vi "Z900_navX_SERIAL_DecodePacket.vi"(8 "error (in)":errorcluster, 10 "Data (in)":u8[](array[numeric]), 11 "Packet (in)":string) -> (0 "error (out)":errorcluster, 1 "empty?":bool, 2 "Data":u8[](array[numeric]), 3 "Packet (out)":string)   [LabVIEW 2016]
uses:
  _TypeDefs/Z900_navX_DeviceRegisters.ctl
  _Util/Encode Protocol/Z900_navX_Util_EncodeProtocol_Int16.vi
  _Util/Z900_navX_Util_BigEndian_to_LittleEndian.vi
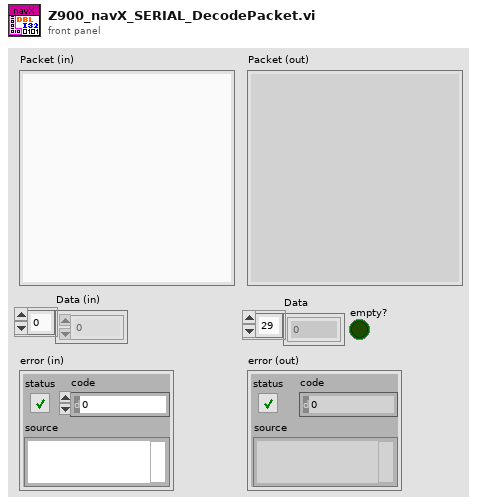
[diagram p1: front panel]
types:
  T1 = typedef "Z900_navX_DeviceRegisters.ctl" = u8
  T2 = cluster{"Device Register":T1, "index":i32, "length":i32}[]
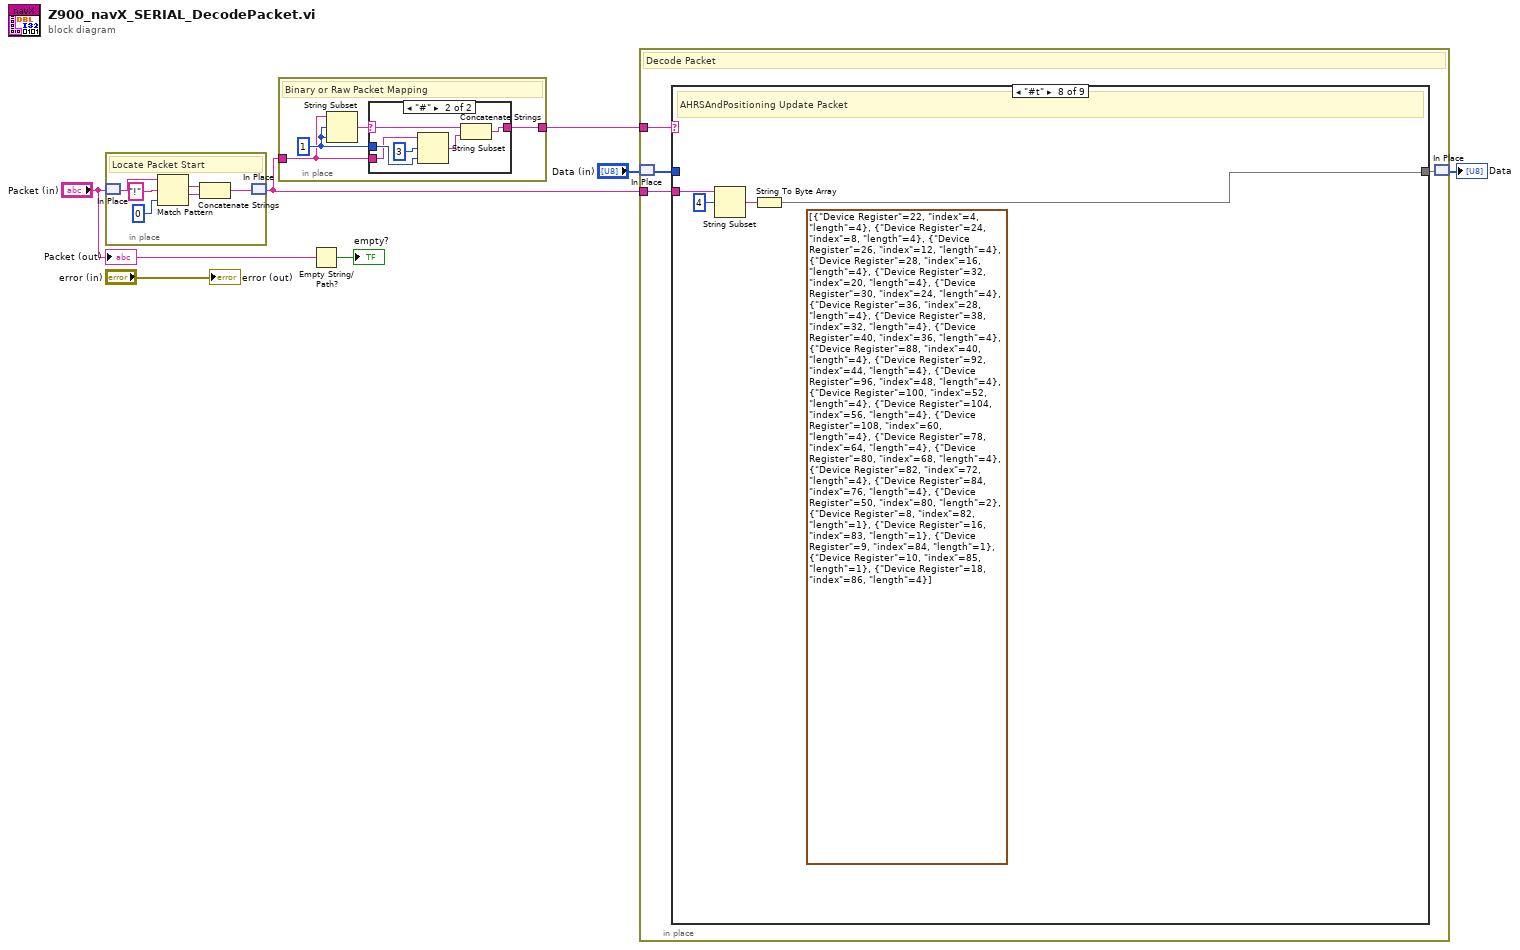
[diagram p0: block diagram]
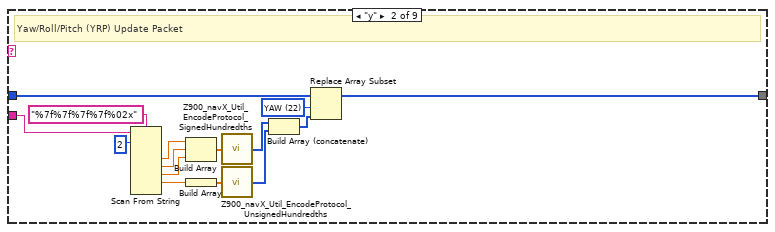
[diagram p3: hidden frame]
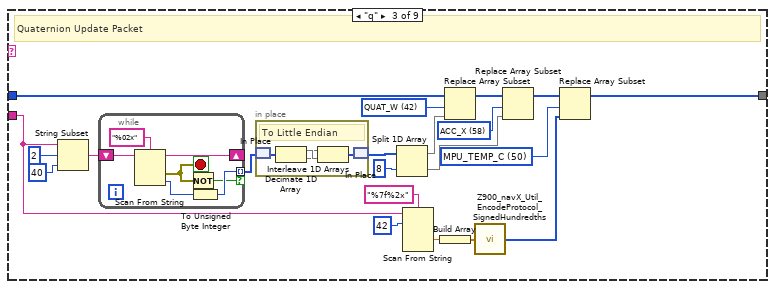
[diagram p4: hidden frame]
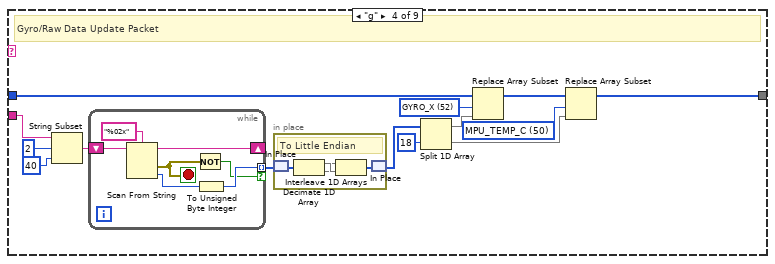
[diagram p5: hidden frame]
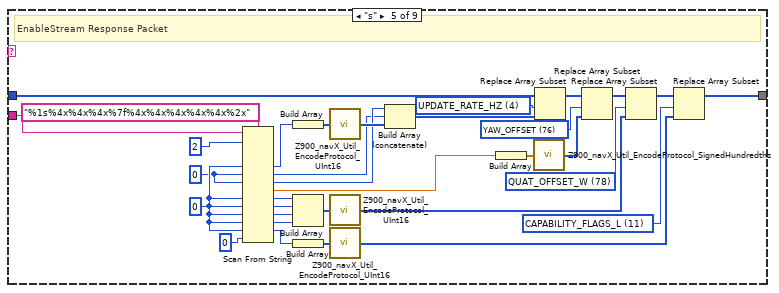
[diagram p6: hidden frame]
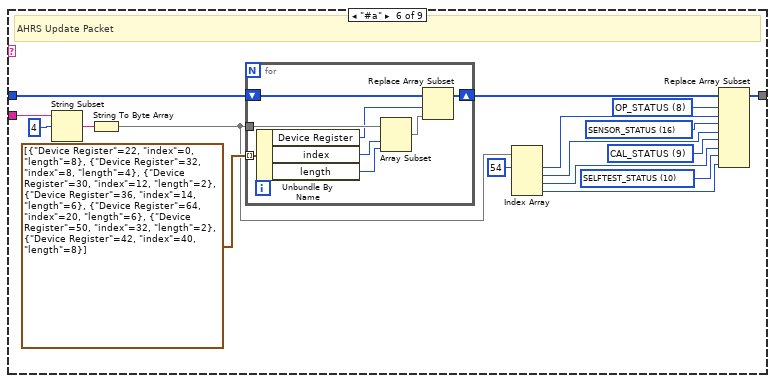
[diagram p7: hidden frame]
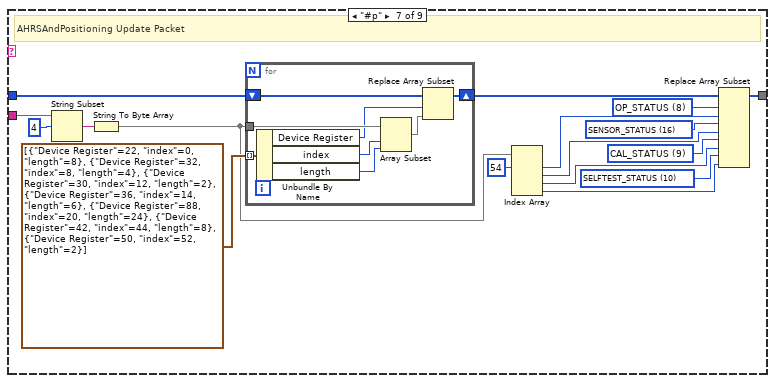
[diagram p8: hidden frame]
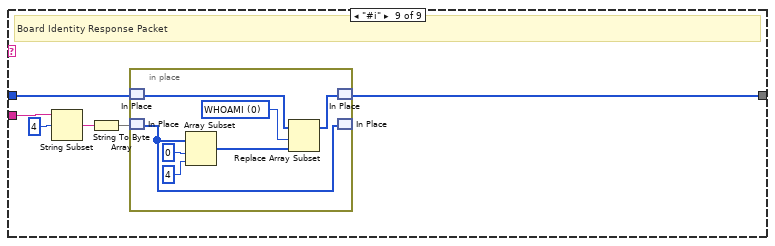
[diagram p9: hidden frame]
diagram:
  n1 = in-place {
    # "Locate Packet Start"
    n2 = in-place-match #1("Packet (in)") -> (w9:string)
    n3 = Match Pattern(string=w9, regular expression="!" ("Packet Start Char"), offset (0)=0 ("offset past match")) -> (match substring=w12:string, after substring=w11:string)  [unwired: 2 out]
    n4 = Concatenate Strings(w12, w11) -> (w8:string)
    n5 = in-place-match #1(w8) -> (w4:string)
  }
  n6 = in-place {
    in-place-border: w4 -> [w15]
    in-place-border: [w17] -> w5
    w16 = 1 ("length (rest)")
    # "Binary or Raw Packet Mapping"
    n7 = String Subset(string=w15, offset (0)=w16, length (rest)=w16) -> (substring=w14:string)
    n8 = case shown="\"#\"" w14 {
      selector: w14 -> [w18 w19]
      tunnel: [w18 w20] -> w17
      tunnel: w16 -> [_ w23]
      tunnel: w15 -> [_ w22]
      frame Default {
      }
      frame "#" {
        n9 = String Subset(string=w22, offset (0)=3, length (rest)=w23) -> (substring=w21:string)
        n10 = Concatenate Strings(w19, w21) -> (w20:string)
      }
    }
  }
  n11 = Empty String/Path?(string/path="Packet (in)") -> (empty?=→"empty?":bool)
  n12 = in-place {
    in-place-border: w5 -> [w28]
    in-place-border: w4 -> [w26]
    # "Decode Packet"
    n13 = in-place-match #2("Data (in)") -> (w27:u8[])
    n14 = case shown="\"#t\"" w28 {
      tunnel: w27 -> [w29 w35 w49 w86 w123 w137 w162 _ w190]
      tunnel: [w29 w30 w55 w79 w112 w135 w160 w185 w189] -> w25
      tunnel: w26 -> [_ w42 w60 w88 w129 w151 w161 w188 w192]
      frame Default {
        # "Unknown Packet"
      }
      frame "y" {
        w31 = T1 22 items=["WHOAMI"=0, "HW_REV"=1, "FW_VER_MAJOR"=2, "FW_VER_MINOR"=3, "UPDATE_RATE_HZ"=4, "ACCEL_FSR_G"=5, "GYRO_FSR_DPS"=6, "OP_STATUS"=8, "CAL_STATUS"=9, "SELFTEST_STATUS"=10, "CAPABILITY_FLAGS_L"=11, "CAPABILITY_FLAGS_H"=12, "SENSOR_STATUS"=16, "TIMESTAMP"=18, "YAW"=22, "ROLL"=24, "PITCH"=26, "HEADING"=28, "FUSED_HEADING"=30, "ALTITUDE_I"=32, "ALTITUDE_D"=34, "LINERA_ACC_X"=36, "LINERA_ACC_Y"=38, "LINERA_ACC_Z"=40, "QUAT_W"=42, "QUAT_X"=44, "QUAT_Y"=46, "QUAT_Z"=48, "MPU_TEMP_C"=50, "GYRO_X"=52, "GYRO_Y"=54, "GYRO_Z"=56, "ACC_X"=58, "ACC_Y"=60, "ACC_Z"=62, "MAG_X"=64, "MAG_Y"=66, "MAG_Z"=68, "PRESSURE_I"=70, "PRESSURE_D"=72, "PRESSURE_TEMP"=74, "YAW_OFFSET"=76, "QUAT_OFFSET_W"=78, "QUAT_OFFSET_X"=80, "QUAT_OFFSET_Y"=82, "QUAT_OFFSET_Z"=84, "INTEGRATION_CONTROL"=86, "VELOCITY_X"=88, "VELOCITY_Y"=92, "VELOCITY_Z"=96, "DISPLACMENT_X"=100, "DISPLACMENT_Y"=104, "DISPLACEMENT_Z"=108] ("Device Register")
        # "Yaw/Roll/Pitch (YRP) Update Packet"
        n15 = Scan From String(format string="%7f%7f%7f%7f%02x", input string=w42, initial scan location=2 ("offset (0)")) -> (output 1=w41:dbl, output 2=w40:dbl, output 3=w39:dbl, output 4=w37:dbl)  [unwired: 7 in, 3 out]
        n16 = Build Array(w41, w40, w39) -> (w38:dbl[])
        n17 = Build Array(w37) -> (w36:dbl[])
        n18 = call "Z900_navX_Util_EncodeProtocol_SignedHundredths.vi"("Signed Hundredths (0.00)"=w38) -> ("Little Endian"=w34:u8[])
        n19 = call "Z900_navX_Util_EncodeProtocol_UnsignedHundredths.vi"("Unsigned Hundredths (0.00)"=w36) -> ("Little Endian"=w33:u8[])
        n20 = Build Array (concatenate)(w34, w33) -> (w32:u8[])
        n21 = Replace Array Subset(array=w35, new element=w32, index=w31) -> (w30:u8[])
      }
      frame "q" {
        w45 = T1 42 items=["WHOAMI"=0, "HW_REV"=1, "FW_VER_MAJOR"=2, "FW_VER_MINOR"=3, "UPDATE_RATE_HZ"=4, "ACCEL_FSR_G"=5, "GYRO_FSR_DPS"=6, "OP_STATUS"=8, "CAL_STATUS"=9, "SELFTEST_STATUS"=10, "CAPABILITY_FLAGS_L"=11, "CAPABILITY_FLAGS_H"=12, "SENSOR_STATUS"=16, "TIMESTAMP"=18, "YAW"=22, "ROLL"=24, "PITCH"=26, "HEADING"=28, "FUSED_HEADING"=30, "ALTITUDE_I"=32, "ALTITUDE_D"=34, "LINERA_ACC_X"=36, "LINERA_ACC_Y"=38, "LINERA_ACC_Z"=40, "QUAT_W"=42, "QUAT_X"=44, "QUAT_Y"=46, "QUAT_Z"=48, "MPU_TEMP_C"=50, "GYRO_X"=52, "GYRO_Y"=54, "GYRO_Z"=56, "ACC_X"=58, "ACC_Y"=60, "ACC_Z"=62, "MAG_X"=64, "MAG_Y"=66, "MAG_Z"=68, "PRESSURE_I"=70, "PRESSURE_D"=72, "PRESSURE_TEMP"=74, "YAW_OFFSET"=76, "QUAT_OFFSET_W"=78, "QUAT_OFFSET_X"=80, "QUAT_OFFSET_Y"=82, "QUAT_OFFSET_Z"=84, "INTEGRATION_CONTROL"=86, "VELOCITY_X"=88, "VELOCITY_Y"=92, "VELOCITY_Z"=96, "DISPLACMENT_X"=100, "DISPLACMENT_Y"=104, "DISPLACEMENT_Z"=108] ("Device Register")
        w52 = T1 58 items=["WHOAMI"=0, "HW_REV"=1, "FW_VER_MAJOR"=2, "FW_VER_MINOR"=3, "UPDATE_RATE_HZ"=4, "ACCEL_FSR_G"=5, "GYRO_FSR_DPS"=6, "OP_STATUS"=8, "CAL_STATUS"=9, "SELFTEST_STATUS"=10, "CAPABILITY_FLAGS_L"=11, "CAPABILITY_FLAGS_H"=12, "SENSOR_STATUS"=16, "TIMESTAMP"=18, "YAW"=22, "ROLL"=24, "PITCH"=26, "HEADING"=28, "FUSED_HEADING"=30, "ALTITUDE_I"=32, "ALTITUDE_D"=34, "LINERA_ACC_X"=36, "LINERA_ACC_Y"=38, "LINERA_ACC_Z"=40, "QUAT_W"=42, "QUAT_X"=44, "QUAT_Y"=46, "QUAT_Z"=48, "MPU_TEMP_C"=50, "GYRO_X"=52, "GYRO_Y"=54, "GYRO_Z"=56, "ACC_X"=58, "ACC_Y"=60, "ACC_Z"=62, "MAG_X"=64, "MAG_Y"=66, "MAG_Z"=68, "PRESSURE_I"=70, "PRESSURE_D"=72, "PRESSURE_TEMP"=74, "YAW_OFFSET"=76, "QUAT_OFFSET_W"=78, "QUAT_OFFSET_X"=80, "QUAT_OFFSET_Y"=82, "QUAT_OFFSET_Z"=84, "INTEGRATION_CONTROL"=86, "VELOCITY_X"=88, "VELOCITY_Y"=92, "VELOCITY_Z"=96, "DISPLACMENT_X"=100, "DISPLACMENT_Y"=104, "DISPLACEMENT_Z"=108] ("Device Register")
        w57 = T1 50 items=["WHOAMI"=0, "HW_REV"=1, "FW_VER_MAJOR"=2, "FW_VER_MINOR"=3, "UPDATE_RATE_HZ"=4, "ACCEL_FSR_G"=5, "GYRO_FSR_DPS"=6, "OP_STATUS"=8, "CAL_STATUS"=9, "SELFTEST_STATUS"=10, "CAPABILITY_FLAGS_L"=11, "CAPABILITY_FLAGS_H"=12, "SENSOR_STATUS"=16, "TIMESTAMP"=18, "YAW"=22, "ROLL"=24, "PITCH"=26, "HEADING"=28, "FUSED_HEADING"=30, "ALTITUDE_I"=32, "ALTITUDE_D"=34, "LINERA_ACC_X"=36, "LINERA_ACC_Y"=38, "LINERA_ACC_Z"=40, "QUAT_W"=42, "QUAT_X"=44, "QUAT_Y"=46, "QUAT_Z"=48, "MPU_TEMP_C"=50, "GYRO_X"=52, "GYRO_Y"=54, "GYRO_Z"=56, "ACC_X"=58, "ACC_Y"=60, "ACC_Z"=62, "MAG_X"=64, "MAG_Y"=66, "MAG_Z"=68, "PRESSURE_I"=70, "PRESSURE_D"=72, "PRESSURE_TEMP"=74, "YAW_OFFSET"=76, "QUAT_OFFSET_W"=78, "QUAT_OFFSET_X"=80, "QUAT_OFFSET_Y"=82, "QUAT_OFFSET_Z"=84, "INTEGRATION_CONTROL"=86, "VELOCITY_X"=88, "VELOCITY_Y"=92, "VELOCITY_Z"=96, "DISPLACMENT_X"=100, "DISPLACMENT_Y"=104, "DISPLACEMENT_Z"=108] ("Device Register")
        # "Quaternion Update Packet"
        n22 = String Subset(string=w60, offset (0)=2, length (rest)=40 ("length (rest)")) -> (substring=w62:string)
        n23 = while {
          shift-right: [w74] -> _
          shift-left: w62 -> [w75]
          tunnel: [w72] -> w51 mode=indexing if=w70
          stop <- w71 stop-if-true
          n24 = Scan From String(format string="%02x", input string=w75) -> (remaining string=w74:string, error out=w71:errorcluster, output 1=w73:u32)  [unwired: 3 in, 1 out]
          n25 = Not(x=w71) -> (.not. x?=w70:bool)
          n26 = To Unsigned Byte Integer(number=w73) -> (unsigned 8bit integer=w72:u8)
        }
        n27 = in-place {
          # "To Little Endian"
          n28 = in-place-match #3(w51) -> (w67:u8[])
          n29 = Decimate 1D Array(w67) -> (w69:u8[], w68:u8[])
          n30 = Interleave 1D Arrays(w68, w69) -> (w66:u8[])
          n31 = in-place-match #3(w66) -> (w50:u8[])
        }
        n32 = Split 1D Array(array=w50, index=8) -> (first subarray=w47:u8[], second subarray=w46:u8[])
        n33 = Scan From String(format string="%7f%2x", input string=w60, initial scan location=u32 42) -> (output 1=w58:dbl)  [unwired: 4 in, 3 out]
        n34 = Build Array(w58) -> (w59:dbl[])
        n35 = Replace Array Subset(array=w49, new element=w47, index=w45) -> (w48:u8[])
        n36 = call "Z900_navX_Util_EncodeProtocol_SignedHundredths.vi"("Signed Hundredths (0.00)"=w59) -> ("Little Endian"=w56:u8[])
        n37 = Replace Array Subset(array=w48, new element=w46, index=w52) -> (w53:u8[])
        n38 = Replace Array Subset(array=w53, new element=w56, index=w57) -> (w55:u8[])
      }
      frame "g" {
        w81 = T1 50 items=["WHOAMI"=0, "HW_REV"=1, "FW_VER_MAJOR"=2, "FW_VER_MINOR"=3, "UPDATE_RATE_HZ"=4, "ACCEL_FSR_G"=5, "GYRO_FSR_DPS"=6, "OP_STATUS"=8, "CAL_STATUS"=9, "SELFTEST_STATUS"=10, "CAPABILITY_FLAGS_L"=11, "CAPABILITY_FLAGS_H"=12, "SENSOR_STATUS"=16, "TIMESTAMP"=18, "YAW"=22, "ROLL"=24, "PITCH"=26, "HEADING"=28, "FUSED_HEADING"=30, "ALTITUDE_I"=32, "ALTITUDE_D"=34, "LINERA_ACC_X"=36, "LINERA_ACC_Y"=38, "LINERA_ACC_Z"=40, "QUAT_W"=42, "QUAT_X"=44, "QUAT_Y"=46, "QUAT_Z"=48, "MPU_TEMP_C"=50, "GYRO_X"=52, "GYRO_Y"=54, "GYRO_Z"=56, "ACC_X"=58, "ACC_Y"=60, "ACC_Z"=62, "MAG_X"=64, "MAG_Y"=66, "MAG_Z"=68, "PRESSURE_I"=70, "PRESSURE_D"=72, "PRESSURE_TEMP"=74, "YAW_OFFSET"=76, "QUAT_OFFSET_W"=78, "QUAT_OFFSET_X"=80, "QUAT_OFFSET_Y"=82, "QUAT_OFFSET_Z"=84, "INTEGRATION_CONTROL"=86, "VELOCITY_X"=88, "VELOCITY_Y"=92, "VELOCITY_Z"=96, "DISPLACMENT_X"=100, "DISPLACMENT_Y"=104, "DISPLACEMENT_Z"=108] ("Device Register")
        w85 = T1 52 items=["WHOAMI"=0, "HW_REV"=1, "FW_VER_MAJOR"=2, "FW_VER_MINOR"=3, "UPDATE_RATE_HZ"=4, "ACCEL_FSR_G"=5, "GYRO_FSR_DPS"=6, "OP_STATUS"=8, "CAL_STATUS"=9, "SELFTEST_STATUS"=10, "CAPABILITY_FLAGS_L"=11, "CAPABILITY_FLAGS_H"=12, "SENSOR_STATUS"=16, "TIMESTAMP"=18, "YAW"=22, "ROLL"=24, "PITCH"=26, "HEADING"=28, "FUSED_HEADING"=30, "ALTITUDE_I"=32, "ALTITUDE_D"=34, "LINERA_ACC_X"=36, "LINERA_ACC_Y"=38, "LINERA_ACC_Z"=40, "QUAT_W"=42, "QUAT_X"=44, "QUAT_Y"=46, "QUAT_Z"=48, "MPU_TEMP_C"=50, "GYRO_X"=52, "GYRO_Y"=54, "GYRO_Z"=56, "ACC_X"=58, "ACC_Y"=60, "ACC_Z"=62, "MAG_X"=64, "MAG_Y"=66, "MAG_Z"=68, "PRESSURE_I"=70, "PRESSURE_D"=72, "PRESSURE_TEMP"=74, "YAW_OFFSET"=76, "QUAT_OFFSET_W"=78, "QUAT_OFFSET_X"=80, "QUAT_OFFSET_Y"=82, "QUAT_OFFSET_Z"=84, "INTEGRATION_CONTROL"=86, "VELOCITY_X"=88, "VELOCITY_Y"=92, "VELOCITY_Z"=96, "DISPLACMENT_X"=100, "DISPLACMENT_Y"=104, "DISPLACEMENT_Z"=108] ("Device Register")
        # "Gyro/Raw Data Update Packet"
        n39 = String Subset(string=w88, offset (0)=2, length (rest)=40 ("length (rest)")) -> (substring=w87:string)
        n40 = while {
          shift-right: [w99] -> _
          shift-left: w87 -> [w100]
          tunnel: [w97] -> w78 mode=indexing if=w95
          stop <- w96 stop-if-true
          n41 = Scan From String(format string="%02x", input string=w100) -> (remaining string=w99:string, error out=w96:errorcluster, output 1=w98:u32)  [unwired: 3 in, 1 out]
          n42 = Not(x=w96) -> (.not. x?=w95:bool)
          n43 = To Unsigned Byte Integer(number=w98) -> (unsigned 8bit integer=w97:u8)
        }
        n44 = in-place {
          # "To Little Endian"
          n45 = in-place-match #4(w78) -> (w92:u8[])
          n46 = Decimate 1D Array(w92) -> (w94:u8[], w93:u8[])
          n47 = Interleave 1D Arrays(w93, w94) -> (w91:u8[])
          n48 = in-place-match #4(w91) -> (w77:u8[])
        }
        n49 = Split 1D Array(array=w77, index=18) -> (first subarray=w84:u8[], second subarray=w80:u8[])
        n50 = Replace Array Subset(array=w86, new element=w84, index=w85) -> (w82:u8[])
        n51 = Replace Array Subset(array=w82, new element=w80, index=w81) -> (w79:u8[])
      }
      frame "s" {
        w105 = u8 0 ("default value 2")
        w114 = T1 11 items=["WHOAMI"=0, "HW_REV"=1, "FW_VER_MAJOR"=2, "FW_VER_MINOR"=3, "UPDATE_RATE_HZ"=4, "ACCEL_FSR_G"=5, "GYRO_FSR_DPS"=6, "OP_STATUS"=8, "CAL_STATUS"=9, "SELFTEST_STATUS"=10, "CAPABILITY_FLAGS_L"=11, "CAPABILITY_FLAGS_H"=12, "SENSOR_STATUS"=16, "TIMESTAMP"=18, "YAW"=22, "ROLL"=24, "PITCH"=26, "HEADING"=28, "FUSED_HEADING"=30, "ALTITUDE_I"=32, "ALTITUDE_D"=34, "LINERA_ACC_X"=36, "LINERA_ACC_Y"=38, "LINERA_ACC_Z"=40, "QUAT_W"=42, "QUAT_X"=44, "QUAT_Y"=46, "QUAT_Z"=48, "MPU_TEMP_C"=50, "GYRO_X"=52, "GYRO_Y"=54, "GYRO_Z"=56, "ACC_X"=58, "ACC_Y"=60, "ACC_Z"=62, "MAG_X"=64, "MAG_Y"=66, "MAG_Z"=68, "PRESSURE_I"=70, "PRESSURE_D"=72, "PRESSURE_TEMP"=74, "YAW_OFFSET"=76, "QUAT_OFFSET_W"=78, "QUAT_OFFSET_X"=80, "QUAT_OFFSET_Y"=82, "QUAT_OFFSET_Z"=84, "INTEGRATION_CONTROL"=86, "VELOCITY_X"=88, "VELOCITY_Y"=92, "VELOCITY_Z"=96, "DISPLACMENT_X"=100, "DISPLACMENT_Y"=104, "DISPLACEMENT_Z"=108] ("Device Register")
        w117 = T1 78 items=["WHOAMI"=0, "HW_REV"=1, "FW_VER_MAJOR"=2, "FW_VER_MINOR"=3, "UPDATE_RATE_HZ"=4, "ACCEL_FSR_G"=5, "GYRO_FSR_DPS"=6, "OP_STATUS"=8, "CAL_STATUS"=9, "SELFTEST_STATUS"=10, "CAPABILITY_FLAGS_L"=11, "CAPABILITY_FLAGS_H"=12, "SENSOR_STATUS"=16, "TIMESTAMP"=18, "YAW"=22, "ROLL"=24, "PITCH"=26, "HEADING"=28, "FUSED_HEADING"=30, "ALTITUDE_I"=32, "ALTITUDE_D"=34, "LINERA_ACC_X"=36, "LINERA_ACC_Y"=38, "LINERA_ACC_Z"=40, "QUAT_W"=42, "QUAT_X"=44, "QUAT_Y"=46, "QUAT_Z"=48, "MPU_TEMP_C"=50, "GYRO_X"=52, "GYRO_Y"=54, "GYRO_Z"=56, "ACC_X"=58, "ACC_Y"=60, "ACC_Z"=62, "MAG_X"=64, "MAG_Y"=66, "MAG_Z"=68, "PRESSURE_I"=70, "PRESSURE_D"=72, "PRESSURE_TEMP"=74, "YAW_OFFSET"=76, "QUAT_OFFSET_W"=78, "QUAT_OFFSET_X"=80, "QUAT_OFFSET_Y"=82, "QUAT_OFFSET_Z"=84, "INTEGRATION_CONTROL"=86, "VELOCITY_X"=88, "VELOCITY_Y"=92, "VELOCITY_Z"=96, "DISPLACMENT_X"=100, "DISPLACMENT_Y"=104, "DISPLACEMENT_Z"=108] ("Device Register")
        w120 = T1 76 items=["WHOAMI"=0, "HW_REV"=1, "FW_VER_MAJOR"=2, "FW_VER_MINOR"=3, "UPDATE_RATE_HZ"=4, "ACCEL_FSR_G"=5, "GYRO_FSR_DPS"=6, "OP_STATUS"=8, "CAL_STATUS"=9, "SELFTEST_STATUS"=10, "CAPABILITY_FLAGS_L"=11, "CAPABILITY_FLAGS_H"=12, "SENSOR_STATUS"=16, "TIMESTAMP"=18, "YAW"=22, "ROLL"=24, "PITCH"=26, "HEADING"=28, "FUSED_HEADING"=30, "ALTITUDE_I"=32, "ALTITUDE_D"=34, "LINERA_ACC_X"=36, "LINERA_ACC_Y"=38, "LINERA_ACC_Z"=40, "QUAT_W"=42, "QUAT_X"=44, "QUAT_Y"=46, "QUAT_Z"=48, "MPU_TEMP_C"=50, "GYRO_X"=52, "GYRO_Y"=54, "GYRO_Z"=56, "ACC_X"=58, "ACC_Y"=60, "ACC_Z"=62, "MAG_X"=64, "MAG_Y"=66, "MAG_Z"=68, "PRESSURE_I"=70, "PRESSURE_D"=72, "PRESSURE_TEMP"=74, "YAW_OFFSET"=76, "QUAT_OFFSET_W"=78, "QUAT_OFFSET_X"=80, "QUAT_OFFSET_Y"=82, "QUAT_OFFSET_Z"=84, "INTEGRATION_CONTROL"=86, "VELOCITY_X"=88, "VELOCITY_Y"=92, "VELOCITY_Z"=96, "DISPLACMENT_X"=100, "DISPLACMENT_Y"=104, "DISPLACEMENT_Z"=108] ("Device Register")
        w122 = T1 4 items=["WHOAMI"=0, "HW_REV"=1, "FW_VER_MAJOR"=2, "FW_VER_MINOR"=3, "UPDATE_RATE_HZ"=4, "ACCEL_FSR_G"=5, "GYRO_FSR_DPS"=6, "OP_STATUS"=8, "CAL_STATUS"=9, "SELFTEST_STATUS"=10, "CAPABILITY_FLAGS_L"=11, "CAPABILITY_FLAGS_H"=12, "SENSOR_STATUS"=16, "TIMESTAMP"=18, "YAW"=22, "ROLL"=24, "PITCH"=26, "HEADING"=28, "FUSED_HEADING"=30, "ALTITUDE_I"=32, "ALTITUDE_D"=34, "LINERA_ACC_X"=36, "LINERA_ACC_Y"=38, "LINERA_ACC_Z"=40, "QUAT_W"=42, "QUAT_X"=44, "QUAT_Y"=46, "QUAT_Z"=48, "MPU_TEMP_C"=50, "GYRO_X"=52, "GYRO_Y"=54, "GYRO_Z"=56, "ACC_X"=58, "ACC_Y"=60, "ACC_Z"=62, "MAG_X"=64, "MAG_Y"=66, "MAG_Z"=68, "PRESSURE_I"=70, "PRESSURE_D"=72, "PRESSURE_TEMP"=74, "YAW_OFFSET"=76, "QUAT_OFFSET_W"=78, "QUAT_OFFSET_X"=80, "QUAT_OFFSET_Y"=82, "QUAT_OFFSET_Z"=84, "INTEGRATION_CONTROL"=86, "VELOCITY_X"=88, "VELOCITY_Y"=92, "VELOCITY_Z"=96, "DISPLACMENT_X"=100, "DISPLACMENT_Y"=104, "DISPLACEMENT_Z"=108] ("Device Register")
        w106 = u16 0
        # "EnableStream Response Packet"
        n52 = Scan From String(format string="%1s%4x%4x%4x%7f%4x%4x%4x%4x%4x%2x", input string=w129, initial scan location=u32 2, default 2=w106, default 3=w105, default 4=w105, default 6=w106, default 7=w106, default 8=w106, default 9=w106, default 10=w106, default 11=u8 0) -> (output 2=w107:u16, output 3=w102:u8, output 4=w103:u8, output 5=w131:dbl, output 6=w128:u16, output 7=w127:u16, output 8=w126:u16, output 9=w125:u16, output 10=w111:u16)  [unwired: 5 in, 3 out]
        n53 = Build Array(w107) -> (w104:u16[])
        n54 = Build Array(w128, w127, w126, w125) -> (w124:u16[])
        n55 = Build Array(w111) -> (w110:u16[])
        n56 = call "Z900_navX_Util_EncodeProtocol_UInt16.vi"("UInt16"=w104) -> ("Little Endian"=w109:u8[])
        n57 = call "Z900_navX_Util_EncodeProtocol_UInt16.vi"("UInt16"=w124) -> ("Little Endian"=w116:u8[])
        n58 = call "Z900_navX_Util_EncodeProtocol_UInt16.vi"("UInt16"=w110) -> ("Little Endian"=w113:u8[])
        n59 = Build Array (concatenate)(w103, w102, w109) -> (w108:u8[])
        n60 = Build Array(w131) -> (w130:dbl[])
        n61 = call "Z900_navX_Util_EncodeProtocol_SignedHundredths.vi"("Signed Hundredths (0.00)"=w130) -> ("Little Endian"=w119:u8[])
        n62 = Replace Array Subset(array=w123, new element=w108, index=w122) -> (w121:u8[])
        n63 = Replace Array Subset(array=w121, new element=w119, index=w120) -> (w118:u8[])
        n64 = Replace Array Subset(array=w118, new element=w116, index=w117) -> (w115:u8[])
        n65 = Replace Array Subset(array=w115, new element=w113, index=w114) -> (w112:u8[])
      }
      frame "#a" {
        w146 = T1 10 items=["WHOAMI"=0, "HW_REV"=1, "FW_VER_MAJOR"=2, "FW_VER_MINOR"=3, "UPDATE_RATE_HZ"=4, "ACCEL_FSR_G"=5, "GYRO_FSR_DPS"=6, "OP_STATUS"=8, "CAL_STATUS"=9, "SELFTEST_STATUS"=10, "CAPABILITY_FLAGS_L"=11, "CAPABILITY_FLAGS_H"=12, "SENSOR_STATUS"=16, "TIMESTAMP"=18, "YAW"=22, "ROLL"=24, "PITCH"=26, "HEADING"=28, "FUSED_HEADING"=30, "ALTITUDE_I"=32, "ALTITUDE_D"=34, "LINERA_ACC_X"=36, "LINERA_ACC_Y"=38, "LINERA_ACC_Z"=40, "QUAT_W"=42, "QUAT_X"=44, "QUAT_Y"=46, "QUAT_Z"=48, "MPU_TEMP_C"=50, "GYRO_X"=52, "GYRO_Y"=54, "GYRO_Z"=56, "ACC_X"=58, "ACC_Y"=60, "ACC_Z"=62, "MAG_X"=64, "MAG_Y"=66, "MAG_Z"=68, "PRESSURE_I"=70, "PRESSURE_D"=72, "PRESSURE_TEMP"=74, "YAW_OFFSET"=76, "QUAT_OFFSET_W"=78, "QUAT_OFFSET_X"=80, "QUAT_OFFSET_Y"=82, "QUAT_OFFSET_Z"=84, "INTEGRATION_CONTROL"=86, "VELOCITY_X"=88, "VELOCITY_Y"=92, "VELOCITY_Z"=96, "DISPLACMENT_X"=100, "DISPLACMENT_Y"=104, "DISPLACEMENT_Z"=108] ("Device Register")
        w145 = T1 9 items=["WHOAMI"=0, "HW_REV"=1, "FW_VER_MAJOR"=2, "FW_VER_MINOR"=3, "UPDATE_RATE_HZ"=4, "ACCEL_FSR_G"=5, "GYRO_FSR_DPS"=6, "OP_STATUS"=8, "CAL_STATUS"=9, "SELFTEST_STATUS"=10, "CAPABILITY_FLAGS_L"=11, "CAPABILITY_FLAGS_H"=12, "SENSOR_STATUS"=16, "TIMESTAMP"=18, "YAW"=22, "ROLL"=24, "PITCH"=26, "HEADING"=28, "FUSED_HEADING"=30, "ALTITUDE_I"=32, "ALTITUDE_D"=34, "LINERA_ACC_X"=36, "LINERA_ACC_Y"=38, "LINERA_ACC_Z"=40, "QUAT_W"=42, "QUAT_X"=44, "QUAT_Y"=46, "QUAT_Z"=48, "MPU_TEMP_C"=50, "GYRO_X"=52, "GYRO_Y"=54, "GYRO_Z"=56, "ACC_X"=58, "ACC_Y"=60, "ACC_Z"=62, "MAG_X"=64, "MAG_Y"=66, "MAG_Z"=68, "PRESSURE_I"=70, "PRESSURE_D"=72, "PRESSURE_TEMP"=74, "YAW_OFFSET"=76, "QUAT_OFFSET_W"=78, "QUAT_OFFSET_X"=80, "QUAT_OFFSET_Y"=82, "QUAT_OFFSET_Z"=84, "INTEGRATION_CONTROL"=86, "VELOCITY_X"=88, "VELOCITY_Y"=92, "VELOCITY_Z"=96, "DISPLACMENT_X"=100, "DISPLACMENT_Y"=104, "DISPLACEMENT_Z"=108] ("Device Register")
        w143 = T1 16 items=["WHOAMI"=0, "HW_REV"=1, "FW_VER_MAJOR"=2, "FW_VER_MINOR"=3, "UPDATE_RATE_HZ"=4, "ACCEL_FSR_G"=5, "GYRO_FSR_DPS"=6, "OP_STATUS"=8, "CAL_STATUS"=9, "SELFTEST_STATUS"=10, "CAPABILITY_FLAGS_L"=11, "CAPABILITY_FLAGS_H"=12, "SENSOR_STATUS"=16, "TIMESTAMP"=18, "YAW"=22, "ROLL"=24, "PITCH"=26, "HEADING"=28, "FUSED_HEADING"=30, "ALTITUDE_I"=32, "ALTITUDE_D"=34, "LINERA_ACC_X"=36, "LINERA_ACC_Y"=38, "LINERA_ACC_Z"=40, "QUAT_W"=42, "QUAT_X"=44, "QUAT_Y"=46, "QUAT_Z"=48, "MPU_TEMP_C"=50, "GYRO_X"=52, "GYRO_Y"=54, "GYRO_Z"=56, "ACC_X"=58, "ACC_Y"=60, "ACC_Z"=62, "MAG_X"=64, "MAG_Y"=66, "MAG_Z"=68, "PRESSURE_I"=70, "PRESSURE_D"=72, "PRESSURE_TEMP"=74, "YAW_OFFSET"=76, "QUAT_OFFSET_W"=78, "QUAT_OFFSET_X"=80, "QUAT_OFFSET_Y"=82, "QUAT_OFFSET_Z"=84, "INTEGRATION_CONTROL"=86, "VELOCITY_X"=88, "VELOCITY_Y"=92, "VELOCITY_Z"=96, "DISPLACMENT_X"=100, "DISPLACMENT_Y"=104, "DISPLACEMENT_Z"=108] ("Device Register")
        w140 = T1 8 items=["WHOAMI"=0, "HW_REV"=1, "FW_VER_MAJOR"=2, "FW_VER_MINOR"=3, "UPDATE_RATE_HZ"=4, "ACCEL_FSR_G"=5, "GYRO_FSR_DPS"=6, "OP_STATUS"=8, "CAL_STATUS"=9, "SELFTEST_STATUS"=10, "CAPABILITY_FLAGS_L"=11, "CAPABILITY_FLAGS_H"=12, "SENSOR_STATUS"=16, "TIMESTAMP"=18, "YAW"=22, "ROLL"=24, "PITCH"=26, "HEADING"=28, "FUSED_HEADING"=30, "ALTITUDE_I"=32, "ALTITUDE_D"=34, "LINERA_ACC_X"=36, "LINERA_ACC_Y"=38, "LINERA_ACC_Z"=40, "QUAT_W"=42, "QUAT_X"=44, "QUAT_Y"=46, "QUAT_Z"=48, "MPU_TEMP_C"=50, "GYRO_X"=52, "GYRO_Y"=54, "GYRO_Z"=56, "ACC_X"=58, "ACC_Y"=60, "ACC_Z"=62, "MAG_X"=64, "MAG_Y"=66, "MAG_Z"=68, "PRESSURE_I"=70, "PRESSURE_D"=72, "PRESSURE_TEMP"=74, "YAW_OFFSET"=76, "QUAT_OFFSET_W"=78, "QUAT_OFFSET_X"=80, "QUAT_OFFSET_Y"=82, "QUAT_OFFSET_Z"=84, "INTEGRATION_CONTROL"=86, "VELOCITY_X"=88, "VELOCITY_Y"=92, "VELOCITY_Z"=96, "DISPLACMENT_X"=100, "DISPLACMENT_Y"=104, "DISPLACEMENT_Z"=108] ("Device Register")
        # "AHRS Update Packet"
        n66 = String Subset(string=w151, offset (0)=4) -> (substring=w149:string)  [unwired: 1 in]
        n67 = String To Byte Array(string=w149) -> (unsigned byte array=w136:u8[])
        n68 = for {
          tunnel: w136 -> [w156]
          tunnel: T2 [{"Device Register"=22, "index"=0, "length"=8}, {"Device Register"=32, "index"=8, "length"=4}, {"Device Register"=30, "index"=12, "length"=2}, {"Device Register"=36, "index"=14, "length"=6}, {"Device Register"=64, "index"=20, "length"=6}, {"Device Register"=50, "index"=32, "length"=2}, {"Device Register"=42, "index"=40, "length"=8}] -> [w155] mode=indexing
          shift-right: [w157] -> w139
          shift-left: w137 -> [w158]
          n69 = Unbundle By Name(w155) -> ("Device Register"=w154:T1, "index"=w153:i32, "length"=w152:i32)
          n70 = Array Subset(array=w156, index=w153, length=w152) -> (w159:u8[])
          n71 = Replace Array Subset(array=w158, new element=w159, index=w154) -> (w157:u8[])
        }
        n72 = Index Array(array=w136, index #1=54 ("index")) -> (element #1=w142:u8, element #2=w144:u8, element #3=w147:u8, element #4=w148:u8)  [unwired: 3 in]
        n73 = Replace Array Subset(array=w139, new element #1=w142, index #1=w140, new element #2=w144, index #2=w143, new element #3=w147, index #3=w145, new element #4=w148, index #4=w146) -> (w135:u8[])
      }
      frame "#p" {
        w172 = T1 10 items=["WHOAMI"=0, "HW_REV"=1, "FW_VER_MAJOR"=2, "FW_VER_MINOR"=3, "UPDATE_RATE_HZ"=4, "ACCEL_FSR_G"=5, "GYRO_FSR_DPS"=6, "OP_STATUS"=8, "CAL_STATUS"=9, "SELFTEST_STATUS"=10, "CAPABILITY_FLAGS_L"=11, "CAPABILITY_FLAGS_H"=12, "SENSOR_STATUS"=16, "TIMESTAMP"=18, "YAW"=22, "ROLL"=24, "PITCH"=26, "HEADING"=28, "FUSED_HEADING"=30, "ALTITUDE_I"=32, "ALTITUDE_D"=34, "LINERA_ACC_X"=36, "LINERA_ACC_Y"=38, "LINERA_ACC_Z"=40, "QUAT_W"=42, "QUAT_X"=44, "QUAT_Y"=46, "QUAT_Z"=48, "MPU_TEMP_C"=50, "GYRO_X"=52, "GYRO_Y"=54, "GYRO_Z"=56, "ACC_X"=58, "ACC_Y"=60, "ACC_Z"=62, "MAG_X"=64, "MAG_Y"=66, "MAG_Z"=68, "PRESSURE_I"=70, "PRESSURE_D"=72, "PRESSURE_TEMP"=74, "YAW_OFFSET"=76, "QUAT_OFFSET_W"=78, "QUAT_OFFSET_X"=80, "QUAT_OFFSET_Y"=82, "QUAT_OFFSET_Z"=84, "INTEGRATION_CONTROL"=86, "VELOCITY_X"=88, "VELOCITY_Y"=92, "VELOCITY_Z"=96, "DISPLACMENT_X"=100, "DISPLACMENT_Y"=104, "DISPLACEMENT_Z"=108] ("Device Register")
        w171 = T1 9 items=["WHOAMI"=0, "HW_REV"=1, "FW_VER_MAJOR"=2, "FW_VER_MINOR"=3, "UPDATE_RATE_HZ"=4, "ACCEL_FSR_G"=5, "GYRO_FSR_DPS"=6, "OP_STATUS"=8, "CAL_STATUS"=9, "SELFTEST_STATUS"=10, "CAPABILITY_FLAGS_L"=11, "CAPABILITY_FLAGS_H"=12, "SENSOR_STATUS"=16, "TIMESTAMP"=18, "YAW"=22, "ROLL"=24, "PITCH"=26, "HEADING"=28, "FUSED_HEADING"=30, "ALTITUDE_I"=32, "ALTITUDE_D"=34, "LINERA_ACC_X"=36, "LINERA_ACC_Y"=38, "LINERA_ACC_Z"=40, "QUAT_W"=42, "QUAT_X"=44, "QUAT_Y"=46, "QUAT_Z"=48, "MPU_TEMP_C"=50, "GYRO_X"=52, "GYRO_Y"=54, "GYRO_Z"=56, "ACC_X"=58, "ACC_Y"=60, "ACC_Z"=62, "MAG_X"=64, "MAG_Y"=66, "MAG_Z"=68, "PRESSURE_I"=70, "PRESSURE_D"=72, "PRESSURE_TEMP"=74, "YAW_OFFSET"=76, "QUAT_OFFSET_W"=78, "QUAT_OFFSET_X"=80, "QUAT_OFFSET_Y"=82, "QUAT_OFFSET_Z"=84, "INTEGRATION_CONTROL"=86, "VELOCITY_X"=88, "VELOCITY_Y"=92, "VELOCITY_Z"=96, "DISPLACMENT_X"=100, "DISPLACMENT_Y"=104, "DISPLACEMENT_Z"=108] ("Device Register")
        w169 = T1 16 items=["WHOAMI"=0, "HW_REV"=1, "FW_VER_MAJOR"=2, "FW_VER_MINOR"=3, "UPDATE_RATE_HZ"=4, "ACCEL_FSR_G"=5, "GYRO_FSR_DPS"=6, "OP_STATUS"=8, "CAL_STATUS"=9, "SELFTEST_STATUS"=10, "CAPABILITY_FLAGS_L"=11, "CAPABILITY_FLAGS_H"=12, "SENSOR_STATUS"=16, "TIMESTAMP"=18, "YAW"=22, "ROLL"=24, "PITCH"=26, "HEADING"=28, "FUSED_HEADING"=30, "ALTITUDE_I"=32, "ALTITUDE_D"=34, "LINERA_ACC_X"=36, "LINERA_ACC_Y"=38, "LINERA_ACC_Z"=40, "QUAT_W"=42, "QUAT_X"=44, "QUAT_Y"=46, "QUAT_Z"=48, "MPU_TEMP_C"=50, "GYRO_X"=52, "GYRO_Y"=54, "GYRO_Z"=56, "ACC_X"=58, "ACC_Y"=60, "ACC_Z"=62, "MAG_X"=64, "MAG_Y"=66, "MAG_Z"=68, "PRESSURE_I"=70, "PRESSURE_D"=72, "PRESSURE_TEMP"=74, "YAW_OFFSET"=76, "QUAT_OFFSET_W"=78, "QUAT_OFFSET_X"=80, "QUAT_OFFSET_Y"=82, "QUAT_OFFSET_Z"=84, "INTEGRATION_CONTROL"=86, "VELOCITY_X"=88, "VELOCITY_Y"=92, "VELOCITY_Z"=96, "DISPLACMENT_X"=100, "DISPLACMENT_Y"=104, "DISPLACEMENT_Z"=108] ("Device Register")
        w166 = T1 8 items=["WHOAMI"=0, "HW_REV"=1, "FW_VER_MAJOR"=2, "FW_VER_MINOR"=3, "UPDATE_RATE_HZ"=4, "ACCEL_FSR_G"=5, "GYRO_FSR_DPS"=6, "OP_STATUS"=8, "CAL_STATUS"=9, "SELFTEST_STATUS"=10, "CAPABILITY_FLAGS_L"=11, "CAPABILITY_FLAGS_H"=12, "SENSOR_STATUS"=16, "TIMESTAMP"=18, "YAW"=22, "ROLL"=24, "PITCH"=26, "HEADING"=28, "FUSED_HEADING"=30, "ALTITUDE_I"=32, "ALTITUDE_D"=34, "LINERA_ACC_X"=36, "LINERA_ACC_Y"=38, "LINERA_ACC_Z"=40, "QUAT_W"=42, "QUAT_X"=44, "QUAT_Y"=46, "QUAT_Z"=48, "MPU_TEMP_C"=50, "GYRO_X"=52, "GYRO_Y"=54, "GYRO_Z"=56, "ACC_X"=58, "ACC_Y"=60, "ACC_Z"=62, "MAG_X"=64, "MAG_Y"=66, "MAG_Z"=68, "PRESSURE_I"=70, "PRESSURE_D"=72, "PRESSURE_TEMP"=74, "YAW_OFFSET"=76, "QUAT_OFFSET_W"=78, "QUAT_OFFSET_X"=80, "QUAT_OFFSET_Y"=82, "QUAT_OFFSET_Z"=84, "INTEGRATION_CONTROL"=86, "VELOCITY_X"=88, "VELOCITY_Y"=92, "VELOCITY_Z"=96, "DISPLACMENT_X"=100, "DISPLACMENT_Y"=104, "DISPLACEMENT_Z"=108] ("Device Register")
        # "AHRSAndPositioning Update Packet"
        n74 = String Subset(string=w161, offset (0)=4) -> (substring=w175:string)  [unwired: 1 in]
        n75 = String To Byte Array(string=w175) -> (unsigned byte array=w163:u8[])
        n76 = for {
          tunnel: w163 -> [w181]
          tunnel: T2 [{"Device Register"=22, "index"=0, "length"=8}, {"Device Register"=32, "index"=8, "length"=4}, {"Device Register"=30, "index"=12, "length"=2}, {"Device Register"=36, "index"=14, "length"=6}, {"Device Register"=88, "index"=20, "length"=24}, {"Device Register"=42, "index"=44, "length"=8}, {"Device Register"=50, "index"=52, "length"=2}] -> [w180] mode=indexing
          shift-right: [w182] -> w165
          shift-left: w162 -> [w183]
          n77 = Unbundle By Name(w180) -> ("Device Register"=w179:T1, "index"=w178:i32, "length"=w177:i32)
          n78 = Array Subset(array=w181, index=w178, length=w177) -> (w184:u8[])
          n79 = Replace Array Subset(array=w183, new element=w184, index=w179) -> (w182:u8[])
        }
        n80 = Index Array(array=w163, index #1=54 ("index")) -> (element #1=w168:u8, element #2=w170:u8, element #3=w173:u8, element #4=w174:u8)  [unwired: 3 in]
        n81 = Replace Array Subset(array=w165, new element #1=w168, index #1=w166, new element #2=w170, index #2=w169, new element #3=w173, index #3=w171, new element #4=w174, index #4=w172) -> (w160:u8[])
      }
      frame "#t" {
        (unwired) T2 [{"Device Register"=22, "index"=4, "length"=4}, {"Device Register"=24, "index"=8, "length"=4}, {"Device Register"=26, "index"=12, "length"=4}, {"Device Register"=28, "index"=16, "length"=4}, {"Device Register"=32, "index"=20, "length"=4}, {"Device Register"=30, "index"=24, "length"=4}, {"Device Register"=36, "index"=28, "length"=4}, {"Device Register"=38, "index"=32, "length"=4}, {"Device Register"=40, "index"=36, "length"=4}, {"Device Register"=88, "index"=40, "length"=4}, {"Device Register"=92, "index"=44, "length"=4}, {"Device Register"=96, "index"=48, "length"=4}, {"Device Register"=100, "index"=52, "length"=4}, {"Device Register"=104, "index"=56, "length"=4}, {"Device Register"=108, "index"=60, "length"=4}, {"Device Register"=78, "index"=64, "length"=4}, {"Device Register"=80, "index"=68, "length"=4}, {"Device Register"=82, "index"=72, "length"=4}, {"Device Register"=84, "index"=76, "length"=4}, {"Device Register"=50, "index"=80, "length"=2}, {"Device Register"=8, "index"=82, "length"=1}, {"Device Register"=16, "index"=83, "length"=1}, {"Device Register"=9, "index"=84, "length"=1}, {"Device Register"=10, "index"=85, "length"=1}, {"Device Register"=18, "index"=86, "length"=4}]
        # "AHRSAndPositioning Update Packet"
        n82 = String Subset(string=w188, offset (0)=4) -> (substring=w187:string)  [unwired: 1 in]
        n83 = String To Byte Array(string=w187) -> (unsigned byte array=w185:u8[])
      }
      frame "#i" {
        # "Board Identity Response Packet"
        n84 = String Subset(string=w192, offset (0)=4) -> (substring=w193:string)  [unwired: 1 in]
        n85 = String To Byte Array(string=w193) -> (unsigned byte array=w191:u8[])
        n86 = in-place {
          w199 = T1 0 items=["WHOAMI"=0, "HW_REV"=1, "FW_VER_MAJOR"=2, "FW_VER_MINOR"=3, "UPDATE_RATE_HZ"=4, "ACCEL_FSR_G"=5, "GYRO_FSR_DPS"=6, "OP_STATUS"=8, "CAL_STATUS"=9, "SELFTEST_STATUS"=10, "CAPABILITY_FLAGS_L"=11, "CAPABILITY_FLAGS_H"=12, "SENSOR_STATUS"=16, "TIMESTAMP"=18, "YAW"=22, "ROLL"=24, "PITCH"=26, "HEADING"=28, "FUSED_HEADING"=30, "ALTITUDE_I"=32, "ALTITUDE_D"=34, "LINERA_ACC_X"=36, "LINERA_ACC_Y"=38, "LINERA_ACC_Z"=40, "QUAT_W"=42, "QUAT_X"=44, "QUAT_Y"=46, "QUAT_Z"=48, "MPU_TEMP_C"=50, "GYRO_X"=52, "GYRO_Y"=54, "GYRO_Z"=56, "ACC_X"=58, "ACC_Y"=60, "ACC_Z"=62, "MAG_X"=64, "MAG_Y"=66, "MAG_Z"=68, "PRESSURE_I"=70, "PRESSURE_D"=72, "PRESSURE_TEMP"=74, "YAW_OFFSET"=76, "QUAT_OFFSET_W"=78, "QUAT_OFFSET_X"=80, "QUAT_OFFSET_Y"=82, "QUAT_OFFSET_Z"=84, "INTEGRATION_CONTROL"=86, "VELOCITY_X"=88, "VELOCITY_Y"=92, "VELOCITY_Z"=96, "DISPLACMENT_X"=100, "DISPLACMENT_Y"=104, "DISPLACEMENT_Z"=108] ("Device Register")
          n87 = in-place-match #5(w190) -> (w198:u8[])
          n88 = in-place-match #6(w191) -> (w195:u8[])
          n89 = Array Subset(array=w195, index=0, length=4) -> (w196:u8[])
          n90 = Replace Array Subset(array=w198, new element=w196, index=w199) -> (w197:u8[])
          n91 = in-place-match #5(w197) -> (w189:u8[])
          n92 = in-place-match #6(w195) -> ()  [unwired: 1 out]
        }
      }
    }
    n93 = in-place-match #2(w25) -> (→"Data":u8[])
  }
  "Packet (out)" <- "Packet (in)"
  "error (out)" <- "error (in)"
